vi "Gain Scheduling on Rising and Falling Process Variable.vi"() -> ()   [LabVIEW 2023]
doc: "This example demonstrates how to use a gain scheduling PID controller to control a simulated process. It also shows how to switch between ranges of PID gains on the rising and falling of process variable."
uses:
  <vilib>/addons/control/pid/pid.llb/PID Gain Schedule (DBL).vi
  <vilib>/addons/control/pid/pid.llb/PID (DBL).vi
  <vilib>/addons/control/pid/NI_PID_pid.lvlib
  <vilib>/ptbypt/NI_PtbyPt.lvlib
panel:
  in  "SP1:":dbl(slide)=32.6797385620915 min=0.0 max=0.0 scale=0.0..100.0
  out "MV1:":dbl(slide)=14.713922690048342 scale=-100.0..100.0
  out "PV1:":dbl(slide)=32.905803767261574 scale=0.0..100.0
  out "Process Variability":T1(graph)={"standard deviation"=0.16234963736437302, "Estimated Measurement\nNoise (%)"=1.0}
  out "Controller Output":dbl(graph)=14.713922690048342
  in  "Expected PV Noise":dbl=1.0
  in  "Plant Measurement Noise":dbl(slide)=0.048035031728659666 scale=0.01..5.0 scale format="%#.5f"
  in  "Tab Control":T2(tab)
  in  "Steady-state Gain":T3={"proportional gain (Kc)"=10.0, "integral time (Ti, min)"=0.01, "derivative time (Td, min)"=0.0} {"derivative time (Td, min)" format="%.3f"; "integral time (Ti, min)" format="%.3f"; "proportional gain (Kc)" format="%.3f"}
  in  "Rising Process Value Gains":T4(array[cluster])=[{"current PID gains"={"proportional gain (Kc)"=30.0, "integral time (Ti, min)"=0.008, "derivative time (Td, min)"=0.001}, "max value"=40.0}, {"current PID gains"={"proportional gain (Kc)"=20.0, "integral time (Ti, min)"=0.01, "derivative time (Td, min)"=0.001}, "max value"=70.0}] {"max value" format="%#.2f"; "current PID gains"."derivative time (Td, min)" format="%.3f"; "current PID gains"."integral time (Ti, min)" format="%.3f"; "current PID gains"."proportional gain (Kc)" format="%#.3f"}
  in  "Falling Process Value Gains":T4(array[cluster])=[{"current PID gains"={"proportional gain (Kc)"=100.0, "integral time (Ti, min)"=0.0, "derivative time (Td, min)"=0.0}, "max value"=40.0}, {"current PID gains"={"proportional gain (Kc)"=1200.0, "integral time (Ti, min)"=0.0, "derivative time (Td, min)"=0.0}, "max value"=70.0}] {"max value" format="%#.2f"; "current PID gains"."derivative time (Td, min)" format="%.3f"; "current PID gains"."integral time (Ti, min)" format="%.3f"; "current PID gains"."proportional gain (Kc)" format="%#.3f"}
  out "Process State":u16(ring) items=["Steady-State", "Rising", "Falling"]
  out "Current PID Gains":T3={"proportional gain (Kc)"=10.0, "integral time (Ti, min)"=0.01, "derivative time (Td, min)"=0.0} {"derivative time (Td, min)" format="%.3f"; "integral time (Ti, min)" format="%.3f"; "proportional gain (Kc)" format="%.3f"}
  in  "Stop":bool
  out "Process Variable and Setpoint":cluster{"initial PV":dbl, "SP1:":dbl}(graph)={"initial PV"=32.905803767261574, "SP1:"=32.6797385620915}
  # "Overview: This example demonstrates how to use a gain scheduling PID controller that change between ranges of PID gains on the rising and falling of process variable.\nRequirements: LabVIEW Full Development System\nInstructions:\n1. Run the VI.\n2.Verify that the Process Variable will be rising until the Process Variability is below Expected PV Noise. Afterwards, the process will be in Steady-State. Note: you could need to change this value depending on the noise level.\n3. Change the setpoint to a lower value and notice that the Process will now use the Falling Parameters.\n4. Verify the Gains on the Steady-State, Rising and Falling PV.\n5. Click Stop to stop the VI."
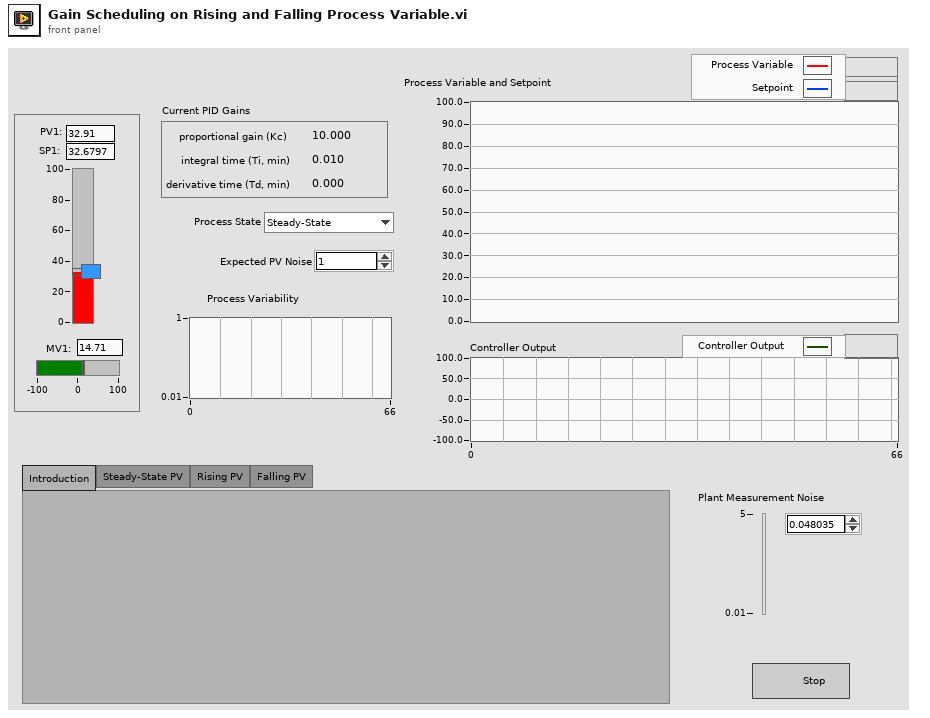
[diagram p1: front panel]
types:
  T1 = cluster{"standard deviation":dbl, "Estimated Measurement\nNoise (%)":dbl}
  T2 = enum32{"Introduction", "Steady-State PV", "Rising PV", "Falling PV"}
  T3 = cluster{"proportional gain (Kc)":dbl, "integral time (Ti, min)":dbl, "derivative time (Td, min)":dbl}
  T4 = cluster{"current PID gains":cluster{"proportional gain (Kc)":dbl, "integral time (Ti, min)":dbl, "derivative time (Td, min)":dbl}, "max value":dbl}[]
  T5 = cluster{"static gain":dbl, "lag (min)":dbl, "dead cycles":dbl, "load %":dbl, "deadband":dbl, "noise level %":dbl, "initial PV":dbl, "initial PV 2":dbl}
  T6 = cluster{"standard deviation":dbl, "Expected PV Noise":dbl}
  T7 = cluster{"Steady-state Gain":cluster{"proportional gain (Kc)":dbl, "integral time (Ti, min)":dbl, "derivative time (Td, min)":dbl}, "x":dbl}
  T8 = cluster{"Steady-state Gain":cluster{"proportional gain (Kc)":dbl, "integral time (Ti, min)":dbl, "derivative time (Td, min)":dbl}, "x":dbl}[]
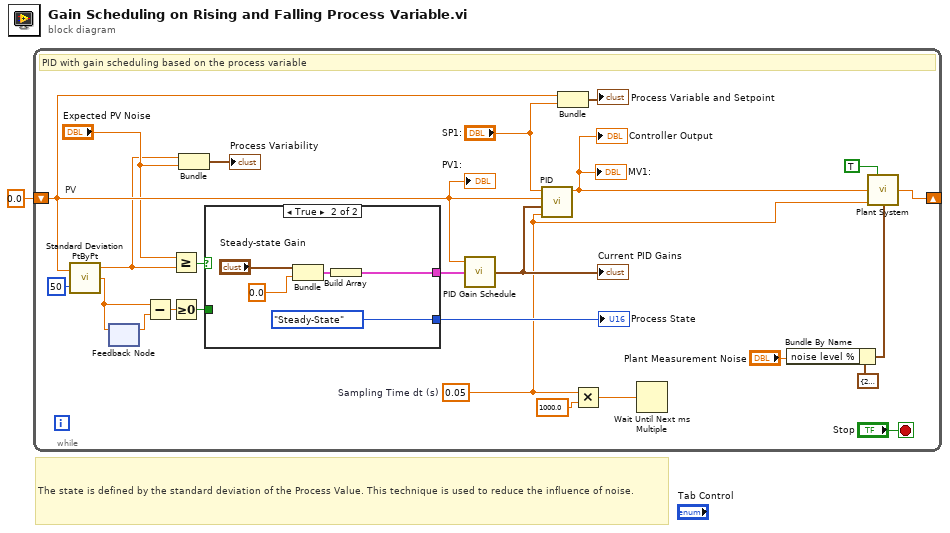
[diagram p0: block diagram]
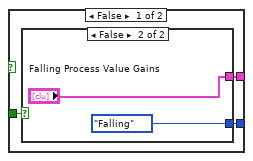
[diagram p2: hidden frame]
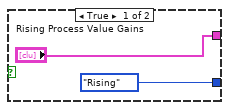
[diagram p3: hidden frame]
diagram:
  # "The state is defined by the standard deviation of the Process Value. This technique is used to reduce the influence of noise."
  n1 = while {
    shift-left: 0.0 ("Plant Output") -> [w15]
    shift-right: [w24] -> _
    stop <- "Stop" stop-if-true
    w2 = 0.05  # Sampling Time dt (s)
    # "PV"
    # "PID with gain scheduling based on the process variable"
    n2 = call <vilib>:"Standard Deviation PtByPt.vi"("x"=w15, "sample length"=50) -> ("standard deviation"=w9:dbl, "mean"=w21:dbl)  [unwired: 1 in, 1 out]
    n3 = feedback-in #1(w21) -> ()
    n4 = feedback #1() -> (w20:dbl)  [unwired: 1 in]
    n5 = Subtract(x=w21, y=w20) -> (x-y=w19:dbl)
    n6 = Greater Or Equal?(x="Expected PV Noise", y=w9) -> (x >= y?=w8:bool)
    n7 = Greater Or Equal To 0?(x=w19) -> (x >= 0?=w17:bool)
    n8 = Bundle("standard deviation"=w9, "Expected PV Noise"="Expected PV Noise") -> (→"Process Variability":T6)  [unwired: 1 in]
    n9 = case shown="True" w8 {
      tunnel: [w28 enum16{"Steady-State", "Rising", "Falling"}."Steady-State" ("Enum")] -> w18
      tunnel: w17 -> [w29 _]
      tunnel: [w27 w34] -> w16
      frame False {
        n10 = case shown="False" w29 {
          tunnel: [enum16{"Steady-State", "Rising", "Falling"}."Rising" ("Enum") enum16{"Steady-State", "Rising", "Falling"}."Falling" ("Enum")] -> w28
          tunnel: ["Rising Process Value Gains" "Falling Process Value Gains"] -> w27
          frame True {
          }
          frame False {
          }
        }
      }
      frame True {
        n11 = Bundle("Steady-state Gain"="Steady-state Gain", "x"=0.0) -> (w35:T7)  [unwired: 1 in]
        n12 = Build Array(w35) -> (w34:T8)
      }
    }
    "Process State" <- w18
    n13 = call-poly <vilib>:"PID Gain Schedule.vi"("PID gain schedule"=w16, "gain scheduling value"=w15) -> ("PID gains out"=w23:T3)  [unwired: 2 in, 1 out]
    "Current PID Gains" <- w23
    n14 = call-poly <vilib>:"PID.vi"("dt (s)"=w2, "PID gains"=w23, "process variable"=w15, "setpoint"="SP1:") -> ("output"=w12:dbl)  [unwired: 6 in, 1 out]
    "MV1:" <- w12
    "Controller Output" <- w12
    n15 = Bundle("Plant Output"=w15, "SP1:"="SP1:") -> (→"Process Variable and Setpoint":cluster{"Plant Output":dbl, "SP1:":dbl})  [unwired: 1 in]
    n16 = Multiply(x=w2, y=1000.0) -> (x*y=w3:dbl)
    n17 = Wait Until Next ms Multiple(millisecond multiple=w3) -> ()  [unwired: 1 out]
    n18 = Bundle By Name(cluster=T5 {"static gain"=2.5, "lag (min)"=18.0, "dead cycles"=0.0, "load %"=40.0, "deadband"=2.0, "noise level %"=0.0, "initial PV"=0.0, "initial PV 2"=0.0} ("process parameters"), "noise level %"="Plant Measurement Noise") -> (w6:T5)
    n19 = call "Plant System.vi"("Integrator ?"=TRUE, "Plant Input"=w12, "dt (s)"=w2, "process parameters"=w6) -> ("Plant Output"=w24:dbl)  [unwired: 11 in]
    "PV1:" <- w15
  }
